vi "TARGET SynchroPhasor DFT NR.vi"() -> ()   [LabVIEW 2014]
uses:
  <vilib>/LabVIEW Targets/FPGA/cRIO/shared/nicrio_ModuleControls/nicrio_cRIO-9467_Altitude.ctl
  <vilib>/LabVIEW Targets/FPGA/cRIO/shared/nicrio_ModuleControls/nicrio_cRIO-9467_Longitude.ctl
  <vilib>/LabVIEW Targets/FPGA/cRIO/shared/nicrio_ModuleControls/nicrio_cRIO-9467_Latitude.ctl
  <vilib>/LabVIEW Targets/FPGA/cRIO/shared/nicrio_ModuleControls/nicrio_cRIO-9227_DataRatesRing.ctl
  <vilib>/LabVIEW Targets/FPGA/cRIO/shared/nicrio_ModuleControls/nicrio_cRIO-9225_DataRatesRing.ctl
  <vilib>/rvi/FXPMathLib/FxpSinAndCos/subVIs/nifxpmath_SinAndCos_SimConfig.ctl
  <vilib>/rvi/FXPMathLib/FxpRectToPolar/subVIs/nifxpmath_RectToPolar_SimConfig.ctl
  <vilib>/rvi/FXPMathLib/FxpDiv/subVIs/nifxpmath_Div_SimConfig.ctl
  <vilib>/rvi/FXPMathLib/FxpPolarToRect/subVIs/nifxpmath_PolarToRect_SimConfig.ctl
  <vilib>/rvi/Emulation/niFpgaGetClockAttributes.vi
  <vilib>/rvi/Emulation/niFpgaSctlEmulationGetInTimedLoop.vi
  <vilib>/rvi/Emulation/niFpgaEmulationReportErrorSimple.vi
  <vilib>/rvi/eio/common/nirviEmuTemplateMethod_errors.vi
  <vilib>/rvi/eio/common/nirviEmuTemplatePropertyGet_noerrors.vi
  <vilib>/rvi/Emulation/niFpgaCriticalErrorInLSC.vi
  <vilib>/rvi/Memory/Memory_Emulation/nirvimemoryFastEmulation.vi
  <vilib>/rvi/Memory/Memory_Emulation/nirvimemoryEmulation.vi
  <vilib>/rvi/Emulation/niFpgaEmulationIsFPGAContextNoSignature.vi
  <vilib>/rvi/DataTransferAndStorage/Container/Common/niFpgaContainerGetUniqueNameForEmu.vi
  <vilib>/rvi/Emulation/niFpgaProcessEmulError.vi
  <vilib>/rvi/errors/nirviReportUnexpectedCaseInternalError (U32).vi
  <vilib>/rvi/FXPMathLib/FxpSinAndCos/simVIs/DllFxpSinAndCosTemp_sub.vi
  <vilib>/rvi/FXPMathLib/FxpRectToPolar/simVIs/DllFxpRectToPolarTemp_sub.vi
  <vilib>/rvi/FXPMathLib/FxpDiv/simVIs/DllFxpDivTemp_sub.vi
  <vilib>/rvi/FXPMathLib/FxpPolarToRect/simVIs/DllFxpPolarToRectTemp_sub.vi
  <vilib>/rvi/DataTransferAndStorage/Container/Common/niFpgaContainerSetEmuInfo.vi
  <vilib>/rvi/eio/common/nirviEmuReportErrorAndStop.vi
  <vilib>/rvi/eio/common/nirviEmuTemplatePropertySet_noerrors.vi
  <vilib>/rvi/eio/common/nirviEmuTemplatePropertyGet_errors.vi
  <vilib>/eio/EIOMethodNode/EIOMethodNode.xnode
  <vilib>/eio/EIOPropertyNode/EIOPropertyNode.xnode
  <vilib>/eio/EIONode/EIONode.xnode
  <vilib>/rvi/DataTransferAndStorage/Container/XNode/niFpgaContainer.xnode
  <vilib>/rvi/FXPMathLib/FxpAdd/XNode/nifxpmath_Add.xnode
  <vilib>/rvi/FXPMathLib/FxpMul/XNode/nifxpmath_Multiplier.xnode
  <vilib>/rvi/FXPMathLib/FxpSinAndCos/XNode/nifxpmath_SinAndCos.xnode
  <vilib>/rvi/FXPMathLib/FxpRectToPolar/XNode/nifxpmath_RectToPolar.xnode
  <vilib>/rvi/FXPMathLib/FxpSub/XNode/nifxpmath_Sub.xnode
  <vilib>/rvi/FXPMathLib/FxpDiv/XNode/nifxpmath_Div.xnode
  <vilib>/rvi/FXPMathLib/FxpPolarToRect/XNode/nifxpmath_PolarToRect.xnode
  <vilib>/rvi/LocalResourceManager/LocalResourceManager.xnode
  <vilib>/rvi/eio/common/nirviEmuTemplatePropertySet_errors.vi
  akhil/fpga timekeeper/FPGA Timekeeper.lvlib
  <vilib>/rvi/FXPMathLib/sim/FxpSim.dll
panel:
  out "Angle Impedance P-G +180":fxp<+/-,24,12>[](array[numeric])
  out "ANGLE P-P +180":fxp<+/-,24,12>[](array[numeric])
  out "ANGLE IMPEDANCE P-G":fxp<+/-,23,11>[](array[numeric])
  out "MAGNITUDE IMOEDANCE P-G":fxp<+,50,25>[](array[numeric])
  out "ANGLE\nIMPEDANCE PHASORS P-P":fxp<+/-,23,11>[](array[numeric])
  out "MAGNITUDE \nIMPEDANCE PHASORS P-P":fxp<+,26,26>[](array[numeric])
  out "IMPEDANCE PHASORS":T1(array[cluster])
  out "ANGLE":fxp<+/-,22,10>[](array[numeric])
  out "PAHSORS":T2(array[cluster])
  out "MAGNITUDE":fxp<+,53,7>[](array[numeric])
  out "Firmware Version":u32 format="%.0x"
  out "Vendor ID":u16 format="%.0x"
  out "Module ID":u16 format="%.0x"
  out "Serial Number":u32 format="%.0x"
  out "FPGA Error Out":errorcluster
  in  "stop 2":bool
  out "PPS Timestamp (TAI)":u64
  out "UTC Offset":i8
  out "UTC Offset Valid":bool
  out "GPS Status":T3(ring)
  out "Antenna Status":T4(ring)
  out "Leap Second Direction":enum8{"Add", "Delete"}(ring)
  out "Leap Second Pending":bool
  out "Leap Second Occurred":bool
  out "Satellites Available":u8
  out "Self-Survey Complete":bool
  out "Latitude (°)":T5 format="%.6f"
  out "Longitude (°)":T6 format="%.6g"
  out "Altitude (m)":T7 format="%.2f"
  out "Timed Out":bool
  out "Iterations":i32
  out "FPGA Timekeeper time (ns)":u64
  out "GPS status":T3(ring)
  out "FPGA Timekeeper locked":bool
  out "offset from time reference":i32
  out "antenna status":T4(ring)
  out "satellites available":u8
  out "UTC offset":i8
  out "UTC offset valid":bool
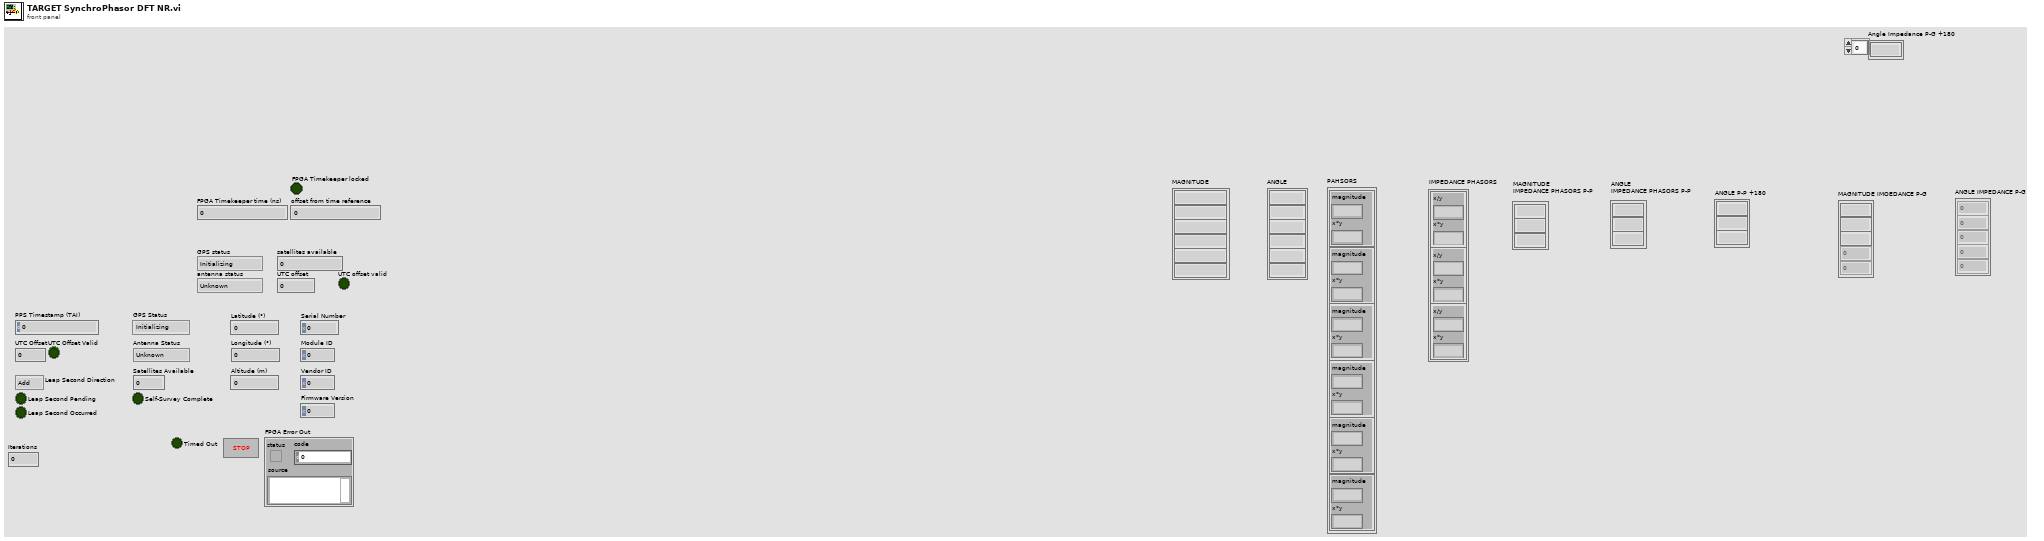
[diagram p1: front panel]
types:
  T1 = cluster{"x/y":fxp<+,26,26>, "x*y":fxp<+/-,23,11>}[]
  T2 = cluster{"magnitude":fxp<+,53,7>, "x*y":fxp<+/-,22,10>}[]
  T3 = enum8{"Initializing", "Normal", "Unable to get fix"}
  T4 = enum8{"Unknown", "Normal", "Absent", "Overcurrent"}
  T5 = typedef "nicrio_cRIO-9467_Latitude.ctl" = fxp<+/-,28,8>
  T6 = typedef "nicrio_cRIO-9467_Longitude.ctl" = fxp<+/-,29,9>
  T7 = typedef "nicrio_cRIO-9467_Altitude.ctl" = fxp<+/-,24,17>
  T8 = typedef "nicrio_cRIO-9225_DataRatesRing.ctl" = u8
  T9 = typedef "nicrio_cRIO-9227_DataRatesRing.ctl" = u8
  T10 = cluster{"magnitude":fxp<+,53,7>, "x*y":fxp<+/-,22,10>}
  T11 = cluster{"x/y":fxp<+,26,26>, "x*y":fxp<+/-,23,11>}
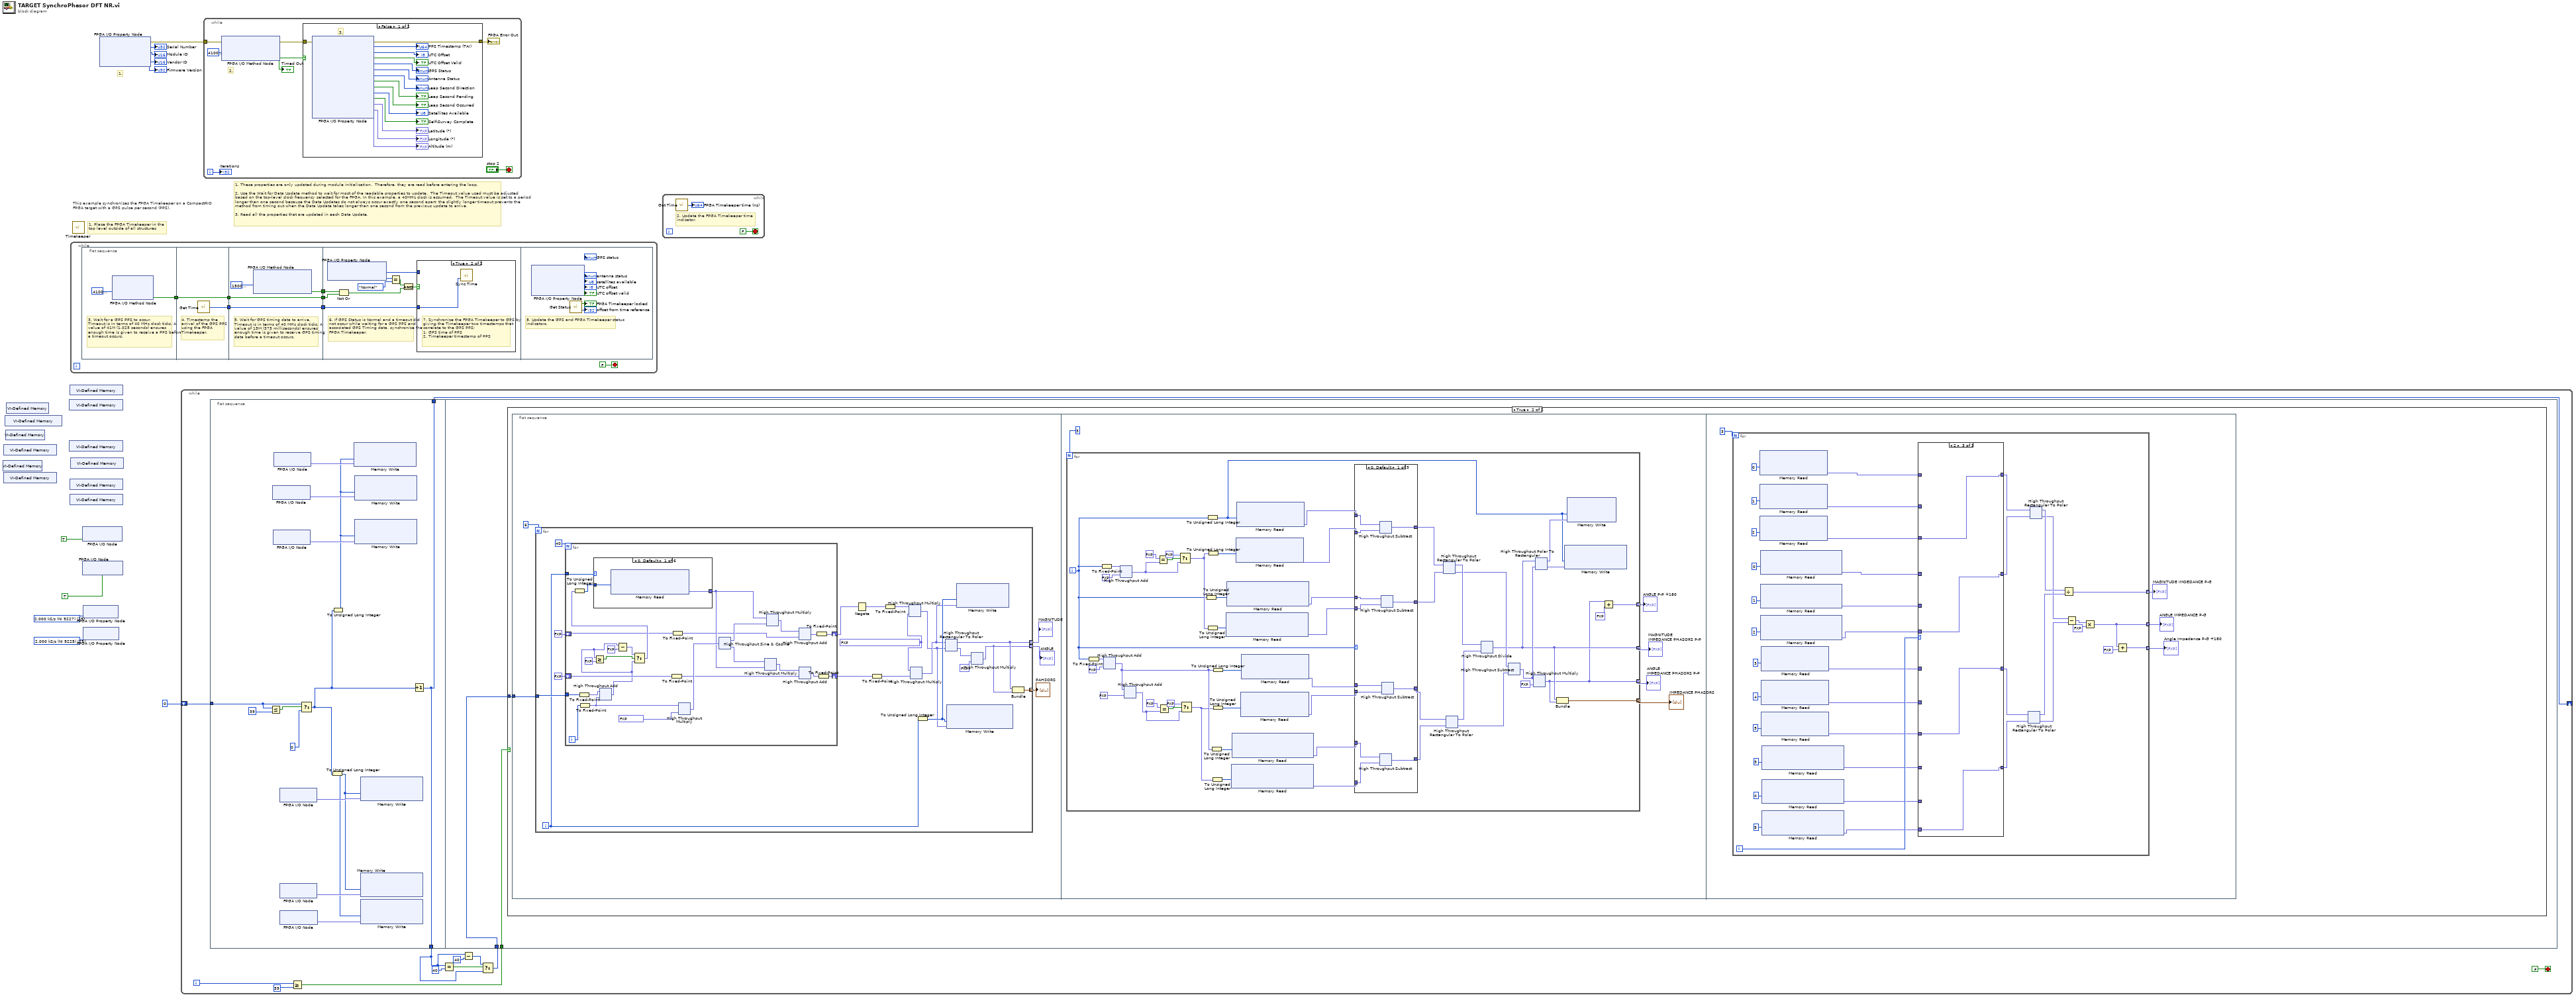
[diagram p0: block diagram]
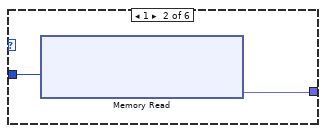
[diagram p3: hidden frame]
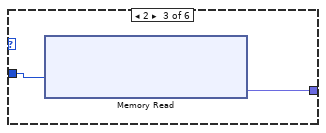
[diagram p4: hidden frame]
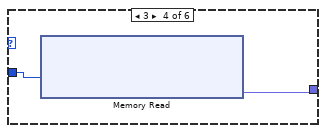
[diagram p5: hidden frame]
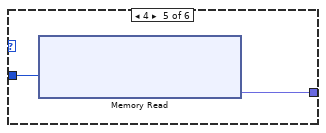
[diagram p6: hidden frame]
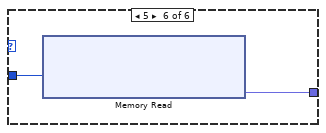
[diagram p7: hidden frame]
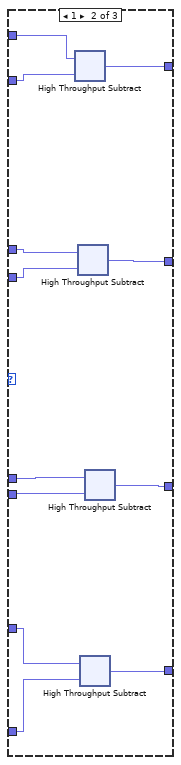
[diagram p8: hidden frame]
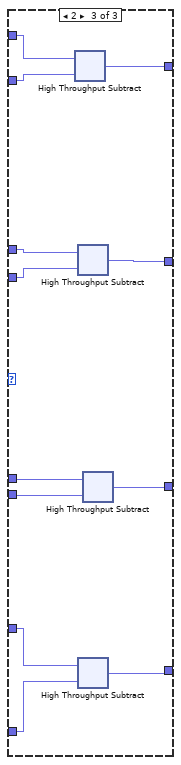
[diagram p9: hidden frame]
diagram:
  w7 = T8 25 items=["50.000 kS/s (NI 9225)"=1, "25.000 kS/s (NI 9225)"=2, "16.667 kS/s (NI 9225)"=3, "12.500 kS/s (NI 9225)"=4, "10.000 kS/s (NI 9225)"=5, "8.333 kS/s (NI 9225)"=6, "7.143 kS/s (NI 9225)"=7, "6.250 kS/s (NI 9225)"=8, "5.556 kS/s (NI 9225)"=9, "5.000 kS/s (NI 9225)"=10, "4.545 kS/s (NI 9225)"=11, "4.167 kS/s (NI 9225)"=12, "3.846 kS/s (NI 9225)"=13, "3.571 kS/s (NI 9225)"=14, "3.333 kS/s (NI 9225)"=15, "3.125 kS/s (NI 9225)"=16, "2.941 kS/s (NI 9225)"=17, "2.778 kS/s (NI 9225)"=18, "2.632 kS/s (NI 9225)"=19, "2.500 kS/s (NI 9225)"=20, "2.381 kS/s (NI 9225)"=21, "2.273 kS/s (NI 9225)"=22, "2.174 kS/s (NI 9225)"=23, "2.083 kS/s (NI 9225)"=24, "2.000 kS/s (NI 9225)"=25, "1.923 kS/s (NI 9225)"=26, "1.852 kS/s (NI 9225)"=27, "1.786 kS/s (NI 9225)"=28, "1.724 kS/s (NI 9225)"=29, "1.667 kS/s (NI 9225)"=30, "1.613 kS/s (NI 9225)"=31] ("Data Rate")
  w8 = T9 25 items=["50.000 kS/s (NI 9227)"=1, "25.000 kS/s (NI 9227)"=2, "16.667 kS/s (NI 9227)"=3, "12.500 kS/s (NI 9227)"=4, "10.000 kS/s (NI 9227)"=5, "8.333 kS/s (NI 9227)"=6, "7.143 kS/s (NI 9227)"=7, "6.250 kS/s (NI 9227)"=8, "5.556 kS/s (NI 9227)"=9, "5.000 kS/s (NI 9227)"=10, "4.545 kS/s (NI 9227)"=11, "4.167 kS/s (NI 9227)"=12, "3.846 kS/s (NI 9227)"=13, "3.571 kS/s (NI 9227)"=14, "3.333 kS/s (NI 9227)"=15, "3.125 kS/s (NI 9227)"=16, "2.941 kS/s (NI 9227)"=17, "2.778 kS/s (NI 9227)"=18, "2.632 kS/s (NI 9227)"=19, "2.500 kS/s (NI 9227)"=20, "2.381 kS/s (NI 9227)"=21, "2.273 kS/s (NI 9227)"=22, "2.174 kS/s (NI 9227)"=23, "2.083 kS/s (NI 9227)"=24, "2.000 kS/s (NI 9227)"=25, "1.923 kS/s (NI 9227)"=26, "1.852 kS/s (NI 9227)"=27, "1.786 kS/s (NI 9227)"=28, "1.724 kS/s (NI 9227)"=29, "1.667 kS/s (NI 9227)"=30, "1.613 kS/s (NI 9227)"=31] ("Data Rate")
  # "1."
  # "1. These properties are only updated during module initialization.  Therefore, they are read before entering the loop.\n\n2. Use the Wait for Data Update method to wait for most of the readable properties to update.  The Timeout value used must be adjusted based on the top-level clock frequency selected for the FPGA. In this example, a 40MHz clock is assumed.  The Timeout value is set to a period longer than one second because the Data Updates do not always occur exactly one second apart; the slightly longer timeout prevents the method from timing out when the Data Update takes longer than one second from the previous update to arrive. \n\n3. Read all the properties that are updated in each Data Update."
  # "This example synchronizes the FPGA Timekeeper on a CompactRIO FPGA target with a GPS pulse per second (PPS)."
  # "1. Place the FPGA Timekeeper in the\ntop level outside of all structures"
  n1 = xnode "VI-Defined Memory"() -> ()  [unwired: 1 out]
  n2 = xnode "VI-Defined Memory"() -> ()  [unwired: 1 out]
  n3 = xnode "VI-Defined Memory"() -> ()  [unwired: 1 out]
  n4 = xnode "VI-Defined Memory"() -> ()  [unwired: 1 out]
  n5 = xnode "VI-Defined Memory"() -> ()  [unwired: 1 out]
  n6 = xnode "VI-Defined Memory"() -> ()  [unwired: 1 out]
  n7 = xnode "VI-Defined Memory"() -> ()  [unwired: 1 out]
  n8 = xnode "VI-Defined Memory"() -> ()  [unwired: 1 out]
  n9 = xnode "VI-Defined Memory"() -> ()  [unwired: 1 out]
  n10 = xnode "VI-Defined Memory"() -> ()  [unwired: 1 out]
  n11 = xnode "VI-Defined Memory"() -> ()  [unwired: 1 out]
  n12 = xnode "VI-Defined Memory"() -> ()  [unwired: 1 out]
  n13 = while {
    stop <- FALSE stop-if-true
    n14 = flat-sequence {
      tunnel: [w19] -> w16
      tunnel: w16 -> [w21]
      tunnel: [w21] -> w15
      tunnel: [w20] -> w13
      tunnel: [w25] -> w17
      tunnel: w15 -> [w24]
      tunnel: [w24] -> w14
      tunnel: w13 -> [w23]
      tunnel: [w23] -> w12
      tunnel: w17 -> [w27]
      tunnel: w14 -> [w26]
      tunnel: w12 -> [w29]
      frame #0 {
        # "3. Wait for a GPS PPS to occur.\nTimeout is in terms of 40 MHz clock ticks. A value of 41M (1.025 seconds) ensures enough time is given to receive a PPS before a timeout occurs."
        n15 = xnode "FPGA I/O Method Node"("Timeout"=41000000) -> ("Timed Out"=w19:bool)  [unwired: 1 in, 1 out]
      }
      frame #1 {
        # "4. Timestamp the arrival of the GPS PPS using the FPGA Timekeeper."
        n16 = call "Get Time.vi"() -> ("time (ns)"=w20:u64)
      }
      frame #2 {
        # "5. Wait for GPS timing data to arrive.\nTimeout is in terms of 40 MHz clock ticks. A value of 15M (375 milliseconds) ensures enough time is given to receive GPS timing data before a timeout occurs."
        n17 = xnode "FPGA I/O Method Node"("Timeout"=15000000) -> ("Timed Out"=w25:bool)  [unwired: 1 in, 1 out]
      }
      frame #3 {
        # "6. If GPS Status is Normal and a timeout did not occur while waiting for a GPS PPS and associated GPS Timing data, synchronize the FPGA Timekeeper."
        n18 = xnode "FPGA I/O Property Node"() -> ("PPS Timestamp (TAI)"=w30:u64, "GPS Status"=w28:T3)  [unwired: 1 in, 1 out]
        n19 = Not Or(1:w26, 2:w27) -> (0:w32:bool)
        n20 = Equal?(x=w28, y=T3."Normal") -> (x = y?=w33:bool)
        n21 = And(x=w33, y=w32) -> (x .and. y?=w31:bool)
        n22 = case shown="True" w31 {
          tunnel: w30 -> [_ _]
          tunnel: w29 -> [_ w35]
          frame False {
          }
          frame True {
            # "7. Synchronize the FPGA Timekeeper to GPS by giving the Timekeeper two timestamps that correlate to the GPS PPS:\n1. GPS time of PPS\n2. Timekeeper timestamp of PPS"
            n23 = call "Sync Time.vi"("FPGA Timekeeper time (ns)"=w35) -> ()  [unwired: 1 in]
          }
        }
      }
      frame #4 {
        # "8. Update the GPS and FPGA Timekeeper status indicators."
        n24 = xnode "FPGA I/O Property Node"() -> ()  [unwired: 1 in, 5 out]
        n25 = call "Get Status.vi"() -> ("FPGA Timekeeper locked"=→"FPGA Timekeeper locked":bool, "offset from time reference"=→"offset from time reference":i32)
      }
    }
  }
  n26 = call "Timekeeper.vi"() -> ()  [unwired: 12 in]
  n27 = xnode "FPGA I/O Node"("Mod3/Start"=TRUE) -> ()  [unwired: 1 in, 1 out]
  n28 = xnode "FPGA I/O Node"("Mod4/Start"=TRUE) -> ()  [unwired: 1 in, 1 out]
  n29 = xnode "FPGA I/O Property Node"("Data Rate"=w8) -> ()  [unwired: 1 in, 1 out]
  n30 = xnode "FPGA I/O Property Node"("Data Rate"=w7) -> ()  [unwired: 1 in, 1 out]
  n31 = xnode "FPGA I/O Property Node"() -> ("error out"=w2:errorcluster, "Serial Number"=→"Serial Number":u32, "Module ID"=→"Module ID":u16, "Vendor ID"=→"Vendor ID":u16, "Firmware Version"=→"Firmware Version":u32)  [unwired: 2 in, 1 out]
  n32 = while {
    shift-right: [w48] -> _
    shift-left: 0 -> [w49]
    i -> [w45]
    stop <- FALSE stop-if-true
    n33 = flat-sequence {
      tunnel: w49 -> [w56]
      tunnel: [w50] -> w48
      tunnel: [w50] -> w38
      tunnel: w47 -> [w65]
      tunnel: w39 -> [w64]
      frame #0 {
        n34 = Less Or Equal?(x=w56, y=39) -> (x <= y?=w57:bool)
        n35 = xnode "FPGA I/O Node"() -> ("Mod4/AI1"=w62:fxp<+/-,24,10>)  [unwired: 1 in, 1 out]
        n36 = xnode "FPGA I/O Node"() -> ("Mod4/AI2"=w61:fxp<+/-,24,10>)  [unwired: 1 in, 1 out]
        n37 = xnode "FPGA I/O Node"() -> ("Mod4/AI0"=w63:fxp<+/-,24,10>)  [unwired: 1 in, 1 out]
        n38 = xnode "FPGA I/O Node"() -> ("Mod3/AI0"=w60:fxp<+/-,24,5>)  [unwired: 1 in, 1 out]
        n39 = xnode "FPGA I/O Node"() -> ("Mod3/AI1"=w59:fxp<+/-,24,5>)  [unwired: 1 in, 1 out]
        n40 = xnode "FPGA I/O Node"() -> ("Mod3/AI2"=w58:fxp<+/-,24,5>)  [unwired: 1 in, 1 out]
        n41 = Select(t=w56, s=w57, f=0) -> (s? t:f=w52:i32)
        n42 = To Unsigned Long Integer(number=w52) -> (unsigned 32bit integer=w51:u32)
        n43 = To Unsigned Long Integer(number=w52) -> (unsigned 32bit integer=w53:u32)
        n44 = xnode ("Memory Write")("Address"=w53, "Data"=w63) -> ()  [unwired: 1 in, 1 out]
        n45 = xnode ("Memory Write")("Address"=w53, "Data"=w62) -> ()  [unwired: 1 in, 1 out]
        n46 = xnode ("Memory Write")("Address"=w53, "Data"=w61) -> ()  [unwired: 1 in, 1 out]
        n47 = xnode ("Memory Write")("Address"=w51, "Data"=w60) -> ()  [unwired: 1 in, 1 out]
        n48 = xnode ("Memory Write")("Address"=w51, "Data"=w59) -> ()  [unwired: 1 in, 1 out]
        n49 = xnode ("Memory Write")("Address"=w51, "Data"=w58) -> ()  [unwired: 1 in, 1 out]
        n50 = Increment(x=w52) -> (x+1=w50:i32)
      }
      frame #1 {
        n51 = case shown="True" w65 {
          tunnel: w64 -> [_ w66]
          frame False {
          }
          frame True {
            n52 = flat-sequence {
              tunnel: w66 -> [w70]
              frame #0 {
                n53 = for {
                  N: 6 -> [_]
                  tunnel: [w81] -> w69 mode=indexing
                  tunnel: [w82] -> w67 mode=indexing
                  tunnel: w70 -> [w85]
                  tunnel: [w80] -> w68 mode=indexing
                  i -> [w79]
                  w86 = fxp<+,28,-4> 0.035355339059606194
                  n54 = for {
                    N: 40 -> [_]
                    tunnel: w79 -> [w147]
                    shift-right: [w128] -> w89
                    shift-left: fxp<+/-,42,14> 0.0 ("x+y") -> [w146]
                    shift-right: [w130] -> w76
                    shift-left: fxp<+/-,42,14> 0.0 ("x+y") -> [w132]
                    tunnel: w85 -> [w141]
                    i -> [w144]
                    n55 = To Fixed-Point(number=w141) -> (fixed-point=w140:fxp<+/-,32,32>)  [unwired: 1 in]
                    n56 = To Fixed-Point(number=w144) -> (fixed-point=w143:fxp<+/-,32,32>)  [unwired: 1 in]
                    n57 = xnode ("High Throughput Add")("x"=w140, "y"=w143) -> ("x+y"=w134:fxp<+/-,33,33>)
                    n58 = Greater Or Equal?(x=w134, y=fxp<+,3,6> 40.0) -> (x >= y?=w138:bool)
                    n59 = Subtract(x=w134, y=fxp<+,3,6> 40.0) -> (x-y=w135:fxp<+/-,34,34>)
                    n60 = Select(t=w135, s=w138, f=w134) -> (s? t:f=w137:fxp<+/-,34,34>)
                    n61 = To Unsigned Long Integer(number=w137) -> (unsigned 32bit integer=w142:u32)
                    n62 = case shown="0, Default" w147 {
                      tunnel: [w186 w188 w190 w192 w194 w196] -> w145
                      tunnel: w142 -> [w185 w187 w189 w191 w193 w195]
                      frame 0, Default {
                        n63 = xnode ("Memory Read")("Address"=w185) -> ("Data"=w186:fxp<+/-,25,11>)  [unwired: 1 in, 1 out]
                      }
                      frame 1 {
                        n64 = xnode ("Memory Read")("Address"=w187) -> ("Data"=w188:fxp<+/-,25,11>)  [unwired: 1 in, 1 out]
                      }
                      frame 2 {
                        n65 = xnode ("Memory Read")("Address"=w189) -> ("Data"=w190:fxp<+/-,25,11>)  [unwired: 1 in, 1 out]
                      }
                      frame 3 {
                        n66 = xnode ("Memory Read")("Address"=w191) -> ("Data"=w192:fxp<+/-,25,11>)  [unwired: 1 in, 1 out]
                      }
                      frame 4 {
                        n67 = xnode ("Memory Read")("Address"=w193) -> ("Data"=w194:fxp<+/-,25,11>)  [unwired: 1 in, 1 out]
                      }
                      frame 5 {
                        n68 = xnode ("Memory Read")("Address"=w195) -> ("Data"=w196:fxp<+/-,25,11>)  [unwired: 1 in, 1 out]
                      }
                    }
                    n69 = To Fixed-Point(number=w146) -> (fixed-point=w149:fxp<+/-,25,11>)  [unwired: 1 in]
                    n70 = To Fixed-Point(number=w132) -> (fixed-point=w129:fxp<+/-,25,11>)  [unwired: 1 in]
                    n71 = xnode ("High Throughput Multiply")("x"=w143, "y"=fxp<+,5,-4> 0.05078125) -> ("x*y"=w152:fxp<+/-,37,28>)
                    n72 = xnode "High Throughput Sine & Cosine"("x (pi)"=w152) -> ("sin(x)"=w153:fxp<+/-,16,2>, "cos(x)"=w154:fxp<+/-,16,2>)
                    n73 = xnode ("High Throughput Multiply")("x"=w154, "y"=w145) -> ("x*y"=w150:fxp<+/-,41,13>)
                    n74 = xnode ("High Throughput Multiply")("x"=w145, "y"=w153) -> ("x*y"=w148:fxp<+/-,41,13>)
                    n75 = xnode ("High Throughput Add")("x"=w148, "y"=w129) -> ("x+y"=w133:fxp<+/-,42,14>)
                    n76 = xnode ("High Throughput Add")("x"=w150, "y"=w149) -> ("x+y"=w131:fxp<+/-,42,14>)
                    n77 = To Fixed-Point(number=w133) -> (fixed-point=w130:fxp<+/-,42,14>)  [unwired: 1 in]
                    n78 = To Fixed-Point(number=w131) -> (fixed-point=w128:fxp<+/-,42,14>)  [unwired: 1 in]
                  }
                  n79 = Negate(x=w76) -> (-x=w88:fxp<+/-,43,15>)
                  n80 = To Fixed-Point(number=w89) -> (fixed-point=w87:fxp<+/-,25,11>)  [unwired: 1 in]
                  n81 = To Fixed-Point(number=w88) -> (fixed-point=w75:fxp<+/-,25,11>)  [unwired: 1 in]
                  n82 = xnode ("High Throughput Multiply")("x"=w75, "y"=w86) -> ("x*y"=w74:fxp<+/-,53,7>)
                  n83 = xnode ("High Throughput Multiply")("x"=w86, "y"=w87) -> ("x*y"=w77:fxp<+/-,53,7>)
                  n84 = To Unsigned Long Integer(number=w79) -> (unsigned 32bit integer=w78:u32)
                  n85 = xnode "High Throughput Rectangular To Polar"("x"=w77, "y"=w74) -> ("magnitude"=w82:fxp<+,53,7>, "phase (pi)"=w83:fxp<+/-,16,2>)
                  n86 = xnode ("Memory Write")("Address"=w78, "Data"=w74) -> ()  [unwired: 1 in, 1 out]
                  n87 = xnode ("Memory Write")("Address"=w78, "Data"=w77) -> ()  [unwired: 1 in, 1 out]
                  n88 = xnode ("High Throughput Multiply")("x"=w83, "y"=fxp<+,6,8> 180.0) -> ("x*y"=w81:fxp<+/-,22,10>)
                  n89 = Bundle("magnitude"=w82, "x*y"=w81) -> (w80:T10)  [unwired: 1 in]
                }
                "ANGLE" <- w69
                "PAHSORS" <- w68
                "MAGNITUDE" <- w67
              }
              frame #1 {
                n90 = for {
                  N: 3 -> [_]
                  tunnel: [w204] -> w200 mode=indexing
                  tunnel: [w205] -> w199 mode=indexing
                  tunnel: [w213] -> w198 mode=indexing
                  tunnel: [w202] -> w197 mode=indexing
                  i -> [w209]
                  n91 = To Fixed-Point(number=w209) -> (fixed-point=w232:fxp<+/-,25,11>)  [unwired: 1 in]
                  n92 = To Fixed-Point(number=w209) -> (fixed-point=w244:fxp<+/-,25,11>)  [unwired: 1 in]
                  n93 = xnode ("High Throughput Add")("x"=w232, "y"=fxp<+,2,2> 3.0) -> ("x+y"=w230:fxp<+/-,26,12>)
                  n94 = xnode ("High Throughput Add")("x"=w244, "y"=fxp<+,1,1> 1.0) -> ("x+y"=w223:fxp<+/-,26,12>)
                  n95 = xnode ("High Throughput Add")("x"=w230, "y"=fxp<+,2,2> 1.0) -> ("x+y"=w220:fxp<+/-,27,13>)
                  n96 = Equal?(x=fxp<+,2,2> 3.0 ("y"), y=w223) -> (x = y?=w225:bool)
                  n97 = Equal?(x=fxp<+,2,3> 6.0 ("y"), y=w220) -> (x = y?=w222:bool)
                  n98 = Select(t=fxp<+/-,26,12> 0.0, s=w225, f=w223) -> (s? t:f=w226:fxp<+/-,26,12>)
                  n99 = Select(t=fxp<+/-,27,13> 3.0, s=w222, f=w220) -> (s? t:f=w219:fxp<+/-,27,13>)
                  n100 = To Unsigned Long Integer(number=w209) -> (unsigned 32bit integer=w251:u32)
                  n101 = To Unsigned Long Integer(number=w226) -> (unsigned 32bit integer=w248:u32)
                  n102 = To Unsigned Long Integer(number=w209) -> (unsigned 32bit integer=w208:u32)
                  n103 = To Unsigned Long Integer(number=w226) -> (unsigned 32bit integer=w249:u32)
                  n104 = To Unsigned Long Integer(number=w230) -> (unsigned 32bit integer=w239:u32)
                  n105 = To Unsigned Long Integer(number=w219) -> (unsigned 32bit integer=w237:u32)
                  n106 = To Unsigned Long Integer(number=w230) -> (unsigned 32bit integer=w240:u32)
                  n107 = To Unsigned Long Integer(number=w219) -> (unsigned 32bit integer=w238:u32)
                  n108 = xnode ("Memory Read")("Address"=w248) -> ("Data"=w245:fxp<+/-,25,11>)  [unwired: 1 in, 1 out]
                  n109 = xnode ("Memory Read")("Address"=w251) -> ("Data"=w246:fxp<+/-,25,11>)  [unwired: 1 in, 1 out]
                  n110 = xnode ("Memory Read")("Address"=w237) -> ("Data"=w233:fxp<+/-,25,11>)  [unwired: 1 in, 1 out]
                  n111 = xnode ("Memory Read")("Address"=w239) -> ("Data"=w234:fxp<+/-,25,11>)  [unwired: 1 in, 1 out]
                  n112 = xnode ("Memory Read")("Address"=w249) -> ("Data"=w247:fxp<+/-,25,11>)  [unwired: 1 in, 1 out]
                  n113 = xnode ("Memory Read")("Address"=w208) -> ("Data"=w250:fxp<+/-,25,11>)  [unwired: 1 in, 1 out]
                  n114 = xnode ("Memory Read")("Address"=w238) -> ("Data"=w235:fxp<+/-,25,11>)  [unwired: 1 in, 1 out]
                  n115 = xnode ("Memory Read")("Address"=w240) -> ("Data"=w236:fxp<+/-,25,11>)  [unwired: 1 in, 1 out]
                  n116 = case shown="0, Default" w209 {
                    tunnel: w250 -> [w400 w412 w424]
                    tunnel: w247 -> [w399 w411 w423]
                    tunnel: w246 -> [w397 w409 w421]
                    tunnel: w245 -> [w398 w410 w422]
                    tunnel: [w396 w408 w420] -> w242
                    tunnel: [w395 w407 w419] -> w241
                    tunnel: w236 -> [w394 w404 w418]
                    tunnel: w235 -> [w393 w403 w417]
                    tunnel: w234 -> [w392 w406 w416]
                    tunnel: w233 -> [w391 w405 w415]
                    tunnel: [w390 w401 w413] -> w227
                    tunnel: [w389 w402 w414] -> w228
                    frame 0, Default {
                      n117 = xnode "High Throughput Subtract"("x"=w400, "y"=w399) -> ("x-y"=w396:fxp<+/-,26,12>)
                      n118 = xnode "High Throughput Subtract"("x"=w392, "y"=w391) -> ("x-y"=w390:fxp<+/-,26,12>)
                      n119 = xnode "High Throughput Subtract"("x"=w397, "y"=w398) -> ("x-y"=w395:fxp<+/-,26,12>)
                      n120 = xnode "High Throughput Subtract"("x"=w394, "y"=w393) -> ("x-y"=w389:fxp<+/-,26,12>)
                    }
                    frame 1 {
                      n121 = xnode "High Throughput Subtract"("x"=w412, "y"=w411) -> ("x-y"=w408:fxp<+/-,26,12>)
                      n122 = xnode "High Throughput Subtract"("x"=w409, "y"=w410) -> ("x-y"=w407:fxp<+/-,26,12>)
                      n123 = xnode "High Throughput Subtract"("x"=w406, "y"=w405) -> ("x-y"=w401:fxp<+/-,26,12>)
                      n124 = xnode "High Throughput Subtract"("x"=w404, "y"=w403) -> ("x-y"=w402:fxp<+/-,26,12>)
                    }
                    frame 2 {
                      n125 = xnode "High Throughput Subtract"("x"=w424, "y"=w423) -> ("x-y"=w420:fxp<+/-,26,12>)
                      n126 = xnode "High Throughput Subtract"("x"=w421, "y"=w422) -> ("x-y"=w419:fxp<+/-,26,12>)
                      n127 = xnode "High Throughput Subtract"("x"=w416, "y"=w415) -> ("x-y"=w413:fxp<+/-,26,12>)
                      n128 = xnode "High Throughput Subtract"("x"=w418, "y"=w417) -> ("x-y"=w414:fxp<+/-,26,12>)
                    }
                  }
                  n129 = xnode "High Throughput Rectangular To Polar"("x"=w242, "y"=w241) -> ("magnitude"=w218:fxp<+,26,12>, "phase (pi)"=w216:fxp<+/-,16,2>)
                  n130 = xnode "High Throughput Rectangular To Polar"("x"=w228, "y"=w227) -> ("magnitude"=w217:fxp<+,26,12>, "phase (pi)"=w215:fxp<+/-,16,2>)
                  n131 = xnode "High Throughput Divide"("x"=w218, "y"=w217) -> ("x/y"=w205:fxp<+,26,26>)
                  n132 = xnode "High Throughput Subtract"("x"=w216, "y"=w215) -> ("x-y"=w212:fxp<+/-,17,3>)
                  n133 = xnode ("High Throughput Multiply")("x"=w212, "y"=fxp<+,6,8> 180.0) -> ("x*y"=w204:fxp<+/-,23,11>)
                  n134 = xnode "High Throughput Polar To Rectangular"("magnitude"=w205, "phase (pi)"=w212) -> ("x"=w211:fxp<+/-,28,28>, "y"=w210:fxp<+/-,28,28>)
                  n135 = Bundle("x/y"=w205, "x*y"=w204) -> (w213:T11)  [unwired: 1 in]
                  n136 = xnode ("Memory Write")("Address"=w208, "Data"=w210) -> ()  [unwired: 1 in, 1 out]
                  n137 = xnode ("Memory Write")("Address"=w208, "Data"=w211) -> ()  [unwired: 1 in, 1 out]
                  n138 = Add(x=w204, y=fxp<+/-,23,11> 180.0) -> (x+y=w202:fxp<+/-,24,12>)
                }
                "ANGLE\nIMPEDANCE PHASORS P-P" <- w200
                "MAGNITUDE \nIMPEDANCE PHASORS P-P" <- w199
                "IMPEDANCE PHASORS" <- w198
                "ANGLE P-P +180" <- w197
              }
              frame #2 {
                n139 = for {
                  N: 3 -> [_]
                  tunnel: [w440] -> w427 mode=indexing
                  tunnel: [w431] -> w426 mode=indexing
                  tunnel: [w429] -> w425 mode=indexing
                  i -> [w455]
                  n140 = xnode "Memory Read"("Address"=u32 0) -> ("Data"=w454:fxp<+/-,25,11>)  [unwired: 1 in, 1 out]
                  n141 = xnode "Memory Read"("Address"=u32 1) -> ("Data"=w439:fxp<+/-,25,11>)  [unwired: 1 in, 1 out]
                  n142 = xnode "Memory Read"("Address"=u32 2) -> ("Data"=w435:fxp<+/-,25,11>)  [unwired: 1 in, 1 out]
                  n143 = xnode "Memory Read"("Address"=u32 0) -> ("Data"=w453:fxp<+/-,25,11>)  [unwired: 1 in, 1 out]
                  n144 = xnode "Memory Read"("Address"=u32 1) -> ("Data"=w438:fxp<+/-,25,11>)  [unwired: 1 in, 1 out]
                  n145 = xnode "Memory Read"("Address"=u32 2) -> ("Data"=w434:fxp<+/-,25,11>)  [unwired: 1 in, 1 out]
                  n146 = xnode "Memory Read"("Address"=u32 3) -> ("Data"=w452:fxp<+/-,25,11>)  [unwired: 1 in, 1 out]
                  n147 = xnode "Memory Read"("Address"=u32 4) -> ("Data"=w437:fxp<+/-,25,11>)  [unwired: 1 in, 1 out]
                  n148 = xnode "Memory Read"("Address"=u32 5) -> ("Data"=w433:fxp<+/-,25,11>)  [unwired: 1 in, 1 out]
                  n149 = xnode "Memory Read"("Address"=u32 3) -> ("Data"=w451:fxp<+/-,25,11>)  [unwired: 1 in, 1 out]
                  n150 = xnode "Memory Read"("Address"=u32 4) -> ("Data"=w436:fxp<+/-,25,11>)  [unwired: 1 in, 1 out]
                  n151 = xnode "Memory Read"("Address"=u32 5) -> ("Data"=w432:fxp<+/-,25,11>)  [unwired: 1 in, 1 out]
                  n152 = case shown="2" w455 {
                    tunnel: w454 -> [w545 _ _]
                    tunnel: w453 -> [w544 _ _]
                    tunnel: w452 -> [w543 _ _]
                    tunnel: w451 -> [w542 _ _]
                    tunnel: [w545 w549 w553] -> w450
                    tunnel: [w544 w548 w552] -> w449
                    tunnel: [w543 w547 w551] -> w448
                    tunnel: [w542 w546 w550] -> w447
                    tunnel: w439 -> [_ w549 _]
                    tunnel: w438 -> [_ w548 _]
                    tunnel: w437 -> [_ w547 _]
                    tunnel: w436 -> [_ w546 _]
                    tunnel: w435 -> [_ _ w553]
                    tunnel: w434 -> [_ _ w552]
                    tunnel: w433 -> [_ _ w551]
                    tunnel: w432 -> [_ _ w550]
                    frame 0, Default {
                    }
                    frame 1 {
                    }
                    frame 2 {
                    }
                  }
                  n153 = xnode "High Throughput Rectangular To Polar"("x"=w448, "y"=w447) -> ("magnitude"=w445:fxp<+,25,11>, "phase (pi)"=w443:fxp<+/-,16,2>)
                  n154 = xnode "High Throughput Rectangular To Polar"("x"=w450, "y"=w449) -> ("magnitude"=w446:fxp<+,25,11>, "phase (pi)"=w444:fxp<+/-,16,2>)
                  n155 = Divide(x=w446, y=w445) -> (x/y=w440:fxp<+,50,25>)
                  n156 = Subtract(x=w444, y=w443) -> (x-y=w442:fxp<+/-,17,3>)
                  n157 = Multiply(x=w442, y=fxp<+,6,8> 180.0) -> (x*y=w431:fxp<+/-,23,11>)
                  n158 = Add(x=w431, y=fxp<+/-,23,11> 180.0) -> (x+y=w429:fxp<+/-,24,12>)
                }
                "MAGNITUDE IMOEDANCE P-G" <- w427
                "ANGLE IMPEDANCE P-G" <- w426
                "Angle Impedance P-G +180" <- w425
              }
            }
          }
        }
      }
    }
    n159 = Greater Or Equal?(x=w45, y=39) -> (x >= y?=w47:bool)
    n160 = Equal?(x=w38, y=40) -> (x = y?=w42:bool)
    n161 = Subtract(x=w38, y=40) -> (x-y=w41:i32)
    n162 = Select(t=w41, s=w42, f=w38) -> (s? t:f=w39:i32)
  }
  n163 = while {
    tunnel: w2 -> [w555]
    i -> [w554]
    stop <- "stop 2" stop-if-true
    # "2."
    n164 = xnode "FPGA I/O Method Node"("error in"=w555, "Timeout"=41000000) -> ("error out"=w560:errorcluster, "Timed Out"=w557:bool)  [unwired: 1 in, 1 out]
    "Timed Out" <- w557
    n165 = case shown="False" w557 {
      tunnel: w560 -> [w575 w576]
      tunnel: [w564 w576] -> w559
      frame False {
        # "3."
        n166 = xnode "FPGA I/O Property Node"("error in"=w575) -> ("error out"=w564:errorcluster, "PPS Timestamp (TAI)"=→"PPS Timestamp (TAI)":u64, "UTC Offset"=→"UTC Offset":i8, "UTC Offset Valid"=→"UTC Offset Valid":bool, "GPS Status"=→"GPS Status":T3, "Antenna Status"=→"Antenna Status":T4, "Leap Second Direction"=→"Leap Second Direction":enum8{"Add", "Delete"}, "Leap Second Pending"=→"Leap Second Pending":bool, "Leap Second Occurred"=→"Leap Second Occurred":bool, "Satellites Available"=→"Satellites Available":u8, "Self-Survey Complete"=→"Self-Survey Complete":bool, "Latitude (°)"=→"Latitude (°)":T5, "Longitude (°)"=→"Longitude (°)":T6, "Altitude (m)"=→"Altitude (m)":T7)  [unwired: 1 in, 1 out]
      }
      frame True {
      }
    }
    "FPGA Error Out" <- w559
    "Iterations" <- w554
  }
  n167 = while {
    stop <- FALSE stop-if-true
    # "2. Update the FPGA Timekeeper time indicator."
    n168 = call "Get Time.vi"() -> ("time (ns)"=→"FPGA Timekeeper time (ns)":u64)
  }
